vi "Test 5.vi"(8 "error in (no error)":errorcluster, 11 "Test Case In":refnum<class "Tests.lvclass">) -> (0 "error out":errorcluster, 3 "Test Case Out":refnum<class "Tests.lvclass">)   [LabVIEW 2021, in "Tests.lvclass"]
uses:
  Tests.lvclass
  C:/Program Files (x86)/National Instruments/LabVIEW 2021/vi.lib/Astemes/LUnit/Test Case.lvclass
  <vilib>/Astemes/LUnit/Test Case.lvclass/Test Case.ctl
  4993e8ee-a06a-463a-9684-69129f64d5ce.vi
  <vilib>/Astemes/LUnit/Append Pass Result.vi
  <vilib>/Astemes/LUnit/Append Fail Result.vi
  <vilib>/Astemes/LUnit/Describe Comparison.vi
  <vilib>/Astemes/LUnit/Compare Variants.vi
  <vilib>/Astemes/LUnit/Variant to string.vi
  <vilib>/Utility/Data Type/Get Type Information.vi
  <vilib>/Utility/LVClass/Get LV Class Name.vi
  Proto/Board.lvclass
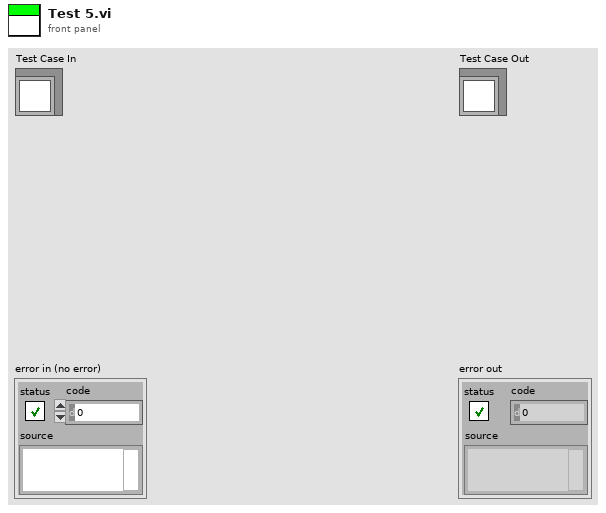
[diagram p1: front panel]
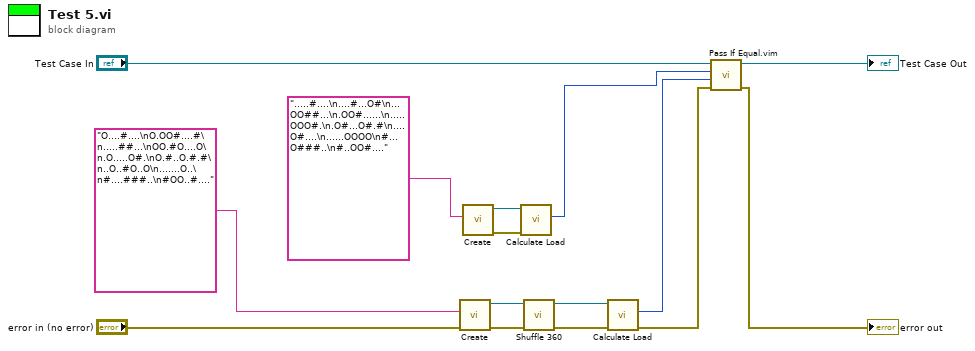
[diagram p0: block diagram]
diagram:
  n1 = call "Create.vi"("error in (no error)"="error in (no error)", "Input"="O....#....\nO.OO#....#\n.....##...\nOO.#O....O\n.O.....O#.\nO.#..O.#.#\n..O..#O..O\n.......O..\n#....###..\n#OO..#....") -> ("error out"=w11:errorcluster, "Proto"=w10:refnum<class "Board.lvclass">)  [unwired: 8 in]
  n2 = call "Create.vi"("Input"=".....#....\n....#...O#\n...OO##...\n.OO#......\n.....OOO#.\n.O#...O#.#\n....O#....\n......OOOO\n#...O###..\n#..OO#....") -> ("error out"=w4:errorcluster, "Proto"=w2:refnum<class "Board.lvclass">)  [unwired: 9 in]
  n3 = call "Calculate Load.vi"("error in (no error)"=w4, "Proto in"=w2) -> ("Load"=w1:u64)  [unwired: 7 in, 2 out]
  n4 = call "Shuffle 360.vi"("error in (no error)"=w11, "Board in"=w10) -> ("error out"=w8:errorcluster, "Board out"=w6:refnum<class "Board.lvclass">)  [unwired: 8 in]
  n5 = call "Calculate Load.vi"("error in (no error)"=w8, "Proto in"=w6) -> ("error out"=w7:errorcluster, "Load"=w5:u64)  [unwired: 7 in, 1 out]
  n6 = call "Pass If Equal.vim"("error in (no error)"=w7, "Actual"=w5, "Expected"=w1, "LUnit Test Case In"="Test Case In") -> ("error out"=→"error out":errorcluster, "LUnit Test Case Out"=→"Test Case Out":refnum<class "Tests.lvclass">)  [unwired: 6 in]
